vi "Check if Reached Start Pos.vi"(6 "Dir(Fwd=T)":bool, 8 "error in (no error)":errorcluster, 9 "Target Encdr Pos.":i32, 10 "Cur Encoder Value":i32, 11 "Status Byte":u16) -> (0 "error out":errorcluster, 1 "Soft Limit?":bool, 2 "Fault or Limit":bool, 3 "ReachedPos?":bool, 5 "MotionStopped?":bool)   [LabVIEW 2015, in "Tool Module.lvlib"]
uses:
  Tool Module.lvlib
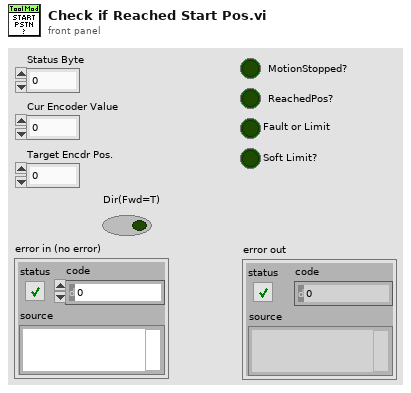
[diagram p1: front panel]
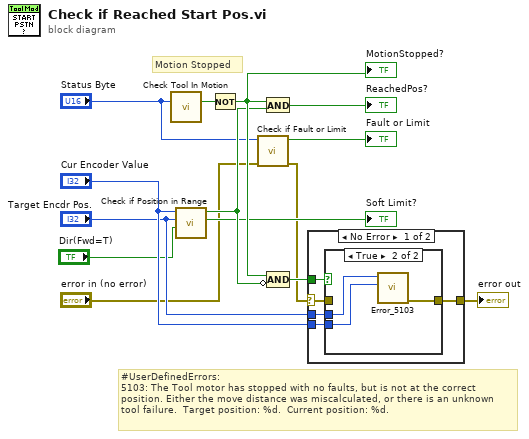
[diagram p0: block diagram]
diagram:
  # "#UserDefinedErrors:\n5103: The Tool motor has stopped with no faults, but is not at the correct position. Either the move distance was miscalculated, or there is an unknown tool failure.  Target position: %d.  Current position: %d."
  # "Motion Stopped"
  n1 = call "Check Tool In Motion.vi"("Status Byte"="Status Byte") -> ("Tool In Motion?"=w14:bool)  [unwired: 14 in]
  n2 = call "Check if Position in Range.vi"("Dir(Fwd=T)"="Dir(Fwd=T)", "Target Position"="Target Encdr Pos.", "Cur Encoder Value"="Cur Encoder Value") -> ("Soft Limit?"=→"Soft Limit?":bool, "In Range?"=w7:bool)  [unwired: 7 in]
  n3 = Not(x=w14) -> (.not. x?=w13:bool)
  "MotionStopped?" <- w13
  n4 = call "Check if Fault or Limit.vi"("error in (no error)"="error in (no error)", "Status In"="Status Byte") -> ("error out"=w3:errorcluster, "Fault or Limit"=→"Fault or Limit":bool)  [unwired: 8 in]
  n5 = And(x=w13, y=w7) -> (x .and. y?=→"ReachedPos?":bool)
  n6 = Compound Arithmetic op=AND(w13, invert w7) -> (w11:bool)
  n7 = case shown="No Error" w3 {
    selector: w3 -> [w18 w24]
    tunnel: w11 -> [w19 _]
    tunnel: [w17 w24] -> w12
    tunnel: "Target Encdr Pos." -> [w16 _]
    tunnel: "Cur Encoder Value" -> [w15 _]
    frame No Error {
      n8 = case shown="True" w19 {
        tunnel: w18 -> [w20 _]
        tunnel: [w20 w21] -> w17
        tunnel: w16 -> [_ w23]
        tunnel: w15 -> [_ w22]
        frame False {
        }
        frame True {
          n9 = call "Error_5103.vi"("Current Pos"=w22, "Target Pos"=w23) -> ("error out"=w21:errorcluster)  [unwired: 9 in]
        }
      }
    }
    frame Error {
    }
  }
  "error out" <- w12
